vi "set_heating_P.vi"(8 "error in (no error)":errorcluster, 10 "P (instr units)":dbl min=-10.0 max=80.0 step=0.1 format="%#.1f", 11 "VISA resource name":refnum<visa-resource-name>) -> (0 "error out":errorcluster, 1 "Unit":string, 2 "P":dbl, 3 "VISA resource name out":refnum<visa-resource-name>)   [LabVIEW 2018]
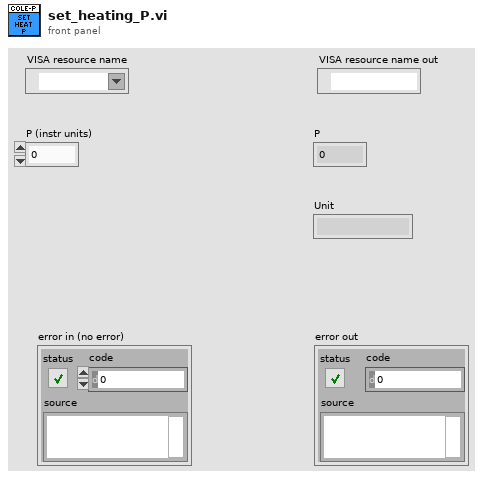
[diagram p1: front panel]
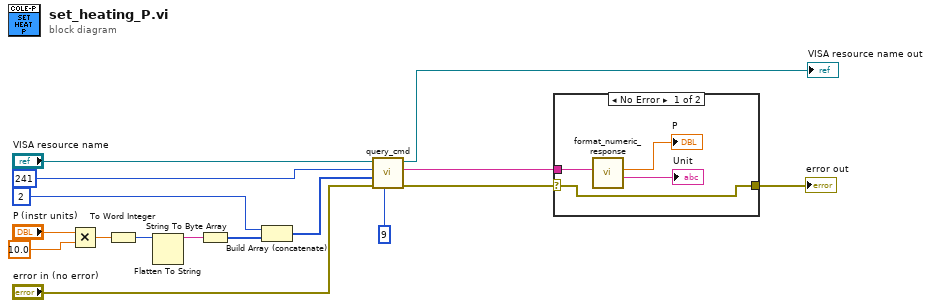
[diagram p0: block diagram]
diagram:
  n1 = Multiply(x="P (instr units)", y=10.0) -> (x*y=w6:dbl)
  n2 = To Word Integer(number=w6) -> (16bit integer=w5:i16)
  n3 = Flatten To String(anything=w5) -> (data string=w4:string)  [unwired: 3 in, 2 out]
  n4 = String To Byte Array(string=w4) -> (unsigned byte array=w3:u8[])
  n5 = Build Array (concatenate)(u8 2, w3) -> (w2:u8[])
  n6 = call "query_cmd.vi"("Number of bytes in response"=u32 9, "error in (no error)"="error in (no error)", "Data bytes"=w2, "Command byte"=u8 241, "VISA resource name"="VISA resource name") -> ("error out"=w10:errorcluster, "Response"=w11:string, "VISA resource name out"=→"VISA resource name out":refnum<visa-resource-name>)  [unwired: 4 in]
  n7 = case shown="No Error" w10 {
    selector: w10 -> [w17 w21]
    tunnel: w11 -> [w20 _]
    tunnel: [w17 w21] -> w9
    frame No Error {
      n8 = call "format_numeric_response.vi"("Response"=w20) -> ("Unit"=→"Unit":string, "Value"=→"P":dbl)  [unwired: 9 in]
    }
    frame Error {
    }
  }
  "error out" <- w9
